vi "Write Parameters.vi"(10 "Parameters":u32[](array[numeric])=[0, 0, 0, 0, 0, 600000, 60000, 100, 3], 11 "HE1_Z_state in":refnum<class "HE_Z_state_v2.lvclass">) -> (3 "HE1_Z_state out":refnum<class "HE_Z_state_v2.lvclass">)   [LabVIEW 2019, in "Heating.lvlib" / "HE_Z_state_v2.lvclass"]
uses:
  HE_Z_state_v2.lvclass
panel:
  # "0 - T_sStop\n1 - T_check"
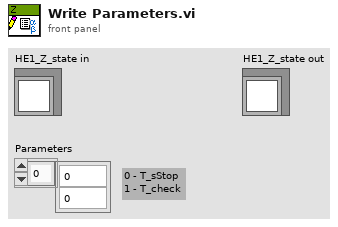
[diagram p1: front panel]
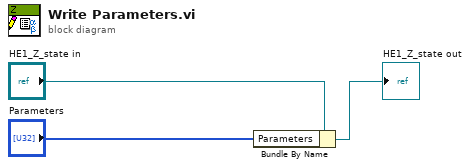
[diagram p0: block diagram]
diagram:
  n1 = Bundle By Name(cluster="HE1_Z_state in", "Parameters"="Parameters") -> (→"HE1_Z_state out":refnum<class "HE_Z_state_v2.lvclass">)
